vi "musicplayer_glo.vi"() -> ()   [LabVIEW 2012]
panel:
  in  "random-data":ext[](array[numeric])
  out "filetypes-snapshot-NOTFOREDIT":string="*.mp3;*.mp4;*.mp2;*.wav;*.wma;*.aifc;*.aiff;*.aif;*.mi;*.snd;*.mid;*.midi;*.cda;*.m4a;*.ogg;*.ts;*.flv;*.asx;*.pl;*.wmv;*.wma;*.m4a;*.m4b"
  in  "titel-info?":bool
  in  "foreground?":bool
  in  "titelname":string
  in  "playing?":bool
  in  "exit?":bool
  in  "Filetypes":string
  in  "random?":bool
  in  "play-alone":bool
  in  "follow-playing-titel?":bool
  out "pfade":string[](array[string])
  in  "stop-event":bool
  in  "new-line-event-main-line":dbl
  in  "new-line-event-main":bool
  in  "play-event-line":dbl=-1.0
  in  "play-event":bool
  in  "playlist sichtbar?":bool
  in  "playlone-lied-Pfad":string
  in  "minimalised?":bool
  in  "overlay?":bool
  in  "main-geschlossen?":bool
  in  "deutsch?":bool
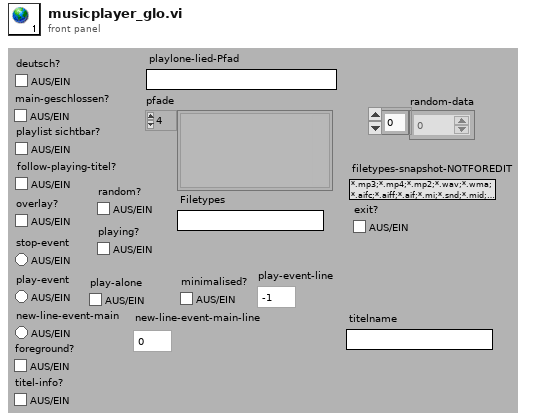
[diagram p1: front panel]
diagram:
